vi "E441X_PM_Initialize.vi"(0 "Instrument Resource Name":refnum<visa-resource-name>="GPIB::13", 5 "ID Query (T: Check)":bool=TRUE, 7 "Reset (T: Reset)":bool=TRUE, 11 "error in (no error)":errorcluster) -> (4 "VISA session":refnum<visa-resource-name>, 15 "error out":errorcluster {"code" format="%.0x"})   [LabVIEW 2015]
doc: "This VI passes the addressing information in the instrument decriptor to the Instr Open VI and returns the instrument ID. You can optionally reset the instrument by setting the front panel reset control. You must run this VI before using any of the instrument driver VIs for this instrument.\n\nNotes:\n(1) This instrument driver supports serial communication. If problems are encountered when using serial communication, it is recommended to try using baud rates less than 19,200 and hardware handshaking. \n\n(2) If you do wish to use the serial interface, set the serial settings on the instrument to be the same as the serial settings on the block diagram and in Measurement & Automation Explorer."
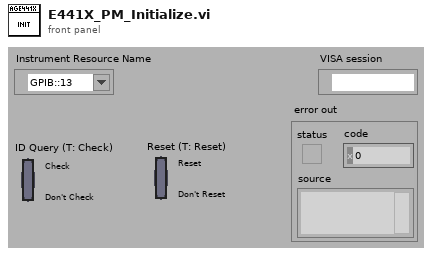
[diagram p1: front panel]
types:
  T1 = cluster{"Status":bool, "Code":i32, "Source (VI Name)":string}
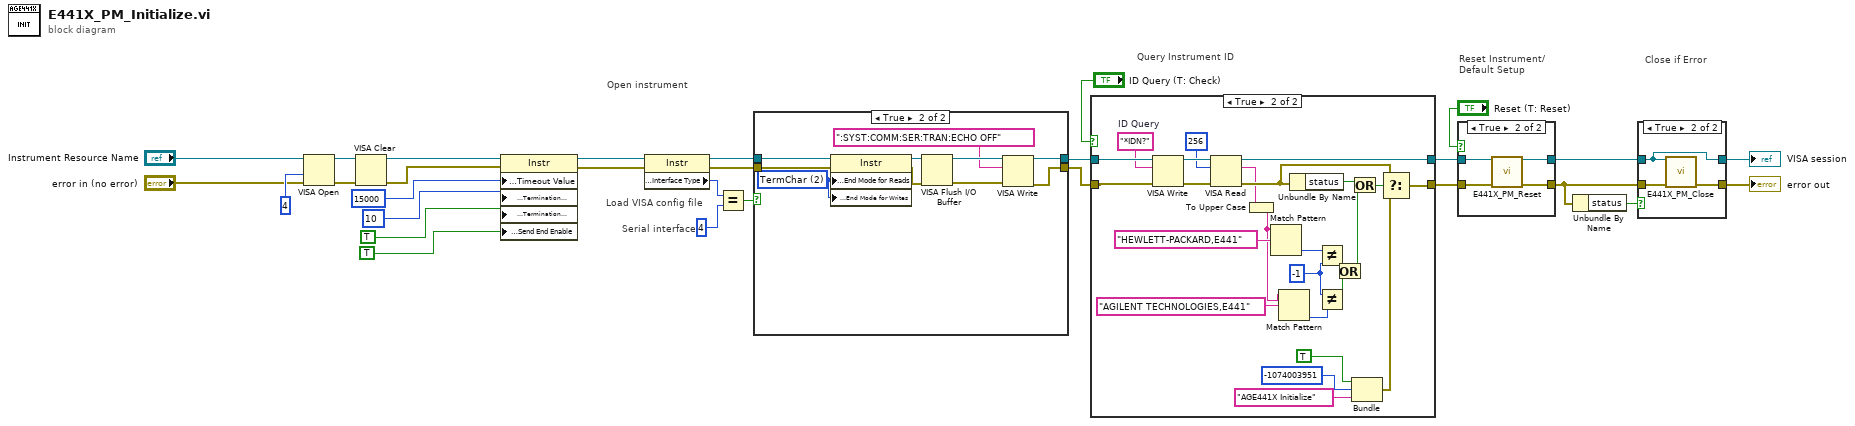
[diagram p0: block diagram]
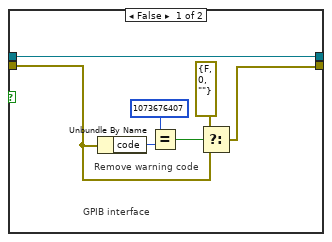
[diagram p2: hidden frame]
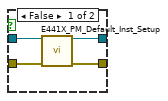
[diagram p4: hidden frame]
diagram:
  # "Serial interface"
  # "Load VISA config file"
  # "Close if Error"
  # "Query Instrument ID"
  # "Reset Instrument/\nDefault Setup"
  # "Open instrument"
  n1 = VISA Open(access mode=u32 4, error in (no error)="error in (no error)", VISA resource name="Instrument Resource Name") -> (VISA resource name=w11:refnum<visa-resource-name>, error out=w12:errorcluster)  [unwired: 2 in]
  n2 = VISA Clear(VISA resource name=w11, error in (no error)=w12) -> (VISA resource name out=w10:refnum<visa-resource-name>, error out=w9:errorcluster)
  n3 = property class="Instr"(reference=w10, error in=w9, "General Settings:Timeout Value"=u32 15000, "Message Based Settings:Termination Character"=u8 10 ("TermChar"), "Message Based Settings:Termination Character Enable"=TRUE ("TermChar En"), "Message Based Settings:Send End Enable"=TRUE) -> (reference out=w4:refnum<visa-resource-name>, error out=w3:errorcluster)
  n4 = property class="Instr"(reference=w4, error in=w3) -> (reference out=w16:refnum<visa-resource-name>, error out=w17:errorcluster, "Interface Information:Interface Type"=w19:u16)
  n5 = Equal?(x=w19, y=u16 4) -> (x = y?=w18:bool)
  n6 = case shown="True" w18 {
    tunnel: w17 -> [w32 w45]
    tunnel: w16 -> [w31 w46]
    tunnel: [w30 w40] -> w14
    tunnel: [w31 w39] -> w13
    frame False {
      # "Remove warning code"
      # "GPIB interface"
      n7 = Unbundle By Name(w32) -> ("code"=w33:i32)
      n8 = Equal?(x=1073676407, y=w33) -> (x = y?=w35:bool)
      n9 = Select(t=errorcluster {"status"=FALSE, "code"=0, "source"=""} ("error out"), s=w35, f=w32) -> (s? t:f=w30:errorcluster)
    }
    frame True {
      w38 = u16 2 items=["None", "LastBit", "TermChar"] ("Serial Settings:Serial End Mode for Reads")
      n10 = property class="Instr"(reference=w46, error in=w45, "Serial Settings:End Mode for Reads"=w38, "Serial Settings:End Mode for Writes"=w38) -> (reference out=w43:refnum<visa-resource-name>, error out=w44:errorcluster)
      n11 = VISA Flush I/O Buffer(VISA resource name=w43, error in (no error)=w44) -> (VISA resource name out=w42:refnum<visa-resource-name>, error out=w41:errorcluster)  [unwired: 1 in]
      n12 = VISA Write(VISA resource name=w42, write buffer=":SYST:COMM:SER:TRAN:ECHO OFF" ("write buffer (\"\")"), error in (no error)=w41) -> (VISA resource name out=w39:refnum<visa-resource-name>, error out=w40:errorcluster)  [unwired: 1 out]
    }
  }
  n13 = case shown="True" "ID Query (T: Check)" {
    tunnel: [w47 w73] -> w28
    tunnel: [w48 w70] -> w29
    tunnel: w13 -> [w48 w71]
    tunnel: w14 -> [w47 w72]
    frame False {
    }
    frame True {
      w61 = "*IDN?"  # ID Query
      w54 = -1
      n14 = VISA Write(VISA resource name=w71, write buffer=w61, error in (no error)=w72) -> (VISA resource name out=w68:refnum<visa-resource-name>, error out=w66:errorcluster)  [unwired: 1 out]
      n15 = VISA Read(VISA resource name=w68, byte count=u32 256, error in (no error)=w66) -> (VISA resource name out=w70:refnum<visa-resource-name>, read buffer=w50:string, error out=w67:errorcluster)  [unwired: 1 out]
      n16 = To Upper Case(1:w50) -> (0:w49:string)
      n17 = Match Pattern(string=w49, regular expression="HEWLETT-PACKARD,E441") -> (offset past match=w55:i32)  [unwired: 1 in, 3 out]
      n18 = Match Pattern(string=w49, regular expression="AGILENT TECHNOLOGIES,E441") -> (offset past match=w56:i32)  [unwired: 1 in, 3 out]
      n19 = Unbundle By Name(w67) -> ("status"=w64:bool)
      n20 = Not Equal?(x=w55, y=w54) -> (x != y?=w52:bool)
      n21 = Not Equal?(x=w54, y=w56) -> (x != y?=w53:bool)
      n22 = Or(x=w52, y=w53) -> (x .or. y?=w51:bool)
      n23 = Or(x=w64, y=w51) -> (x .or. y?=w65:bool)
      n24 = Bundle("Status"=TRUE, "Code"=-1074003951, "Source (VI Name)"="AGE441X Initialize") -> (w60:T1)  [unwired: 1 in]
      n25 = Select(t=w67, s=w65, f=w60) -> (s? t:f=w73:T1)
    }
  }
  n26 = case shown="True" "Reset (T: Reset)" {
    tunnel: w28 -> [w76 w78]
    tunnel: [w75 w81] -> w24
    tunnel: w29 -> [w77 w79]
    tunnel: [w74 w80] -> w23
    frame False {
      n27 = call "E441X_PM_Default_Inst_Setup.vi"("VISA session"=w77, "error in (no error)"=w76) -> ("dup VISA session"=w74:refnum<visa-resource-name>, "error out"=w75:errorcluster)  [unwired: 12 in]
    }
    frame True {
      n28 = call "E441X_PM_Reset.vi"("VISA session"=w79, "error in (no error)"=w78) -> ("dup VISA session"=w80:refnum<visa-resource-name>, "error out"=w81:errorcluster)  [unwired: 12 in]
    }
  }
  n29 = Unbundle By Name(w24) -> ("status"=w25:bool)
  n30 = case shown="True" w25 {
    tunnel: w23 -> [w83 w84]
    tunnel: w24 -> [w82 w86]
    tunnel: [w83 w84] -> w22
    tunnel: [w82 w85] -> w21
    frame False {
    }
    frame True {
      n31 = call "E441X_PM_Close.vi"("VISA session"=w84, "error in (no error)"=w86) -> ("error out"=w85:errorcluster)  [unwired: 13 in]
    }
  }
  "VISA session" <- w22
  "error out" <- w21
